vi "GetServerVIName.vi"(1 "ROS":T1={"topic port"=0, "Node"="", "topic"="", "type"="", "node port"=0, "error "={"status"=FALSE, "code"=0, "source"=""}, "Direction"=enum."Node", "Update (ms)"=1, "FIFO size"=1}) -> (0 "vi name":string)   [LabVIEW 2015]
doc: "Gets VI name"
uses:
  _ROSControl.ctl
  _ROSDirection.ctl
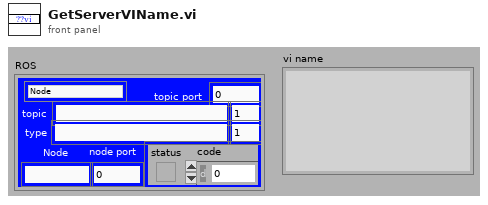
[diagram p1: front panel]
types:
  T1 = typedef "_ROSControl.ctl" = cluster{"topic port":u16, "Node":string, "topic":string, "type":string, "node port":u16, "error ":errorcluster, "Direction":T2, "Update (ms)":u16, "FIFO size":u16}
  T2 = typedef "_ROSDirection.ctl" = enum16{"Node", "Publisher", "Subscriber", "ServiceClient", "ServiceProvider"}
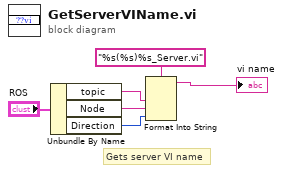
[diagram p0: block diagram]
diagram:
  # "Gets server VI name"
  n1 = Unbundle By Name("ROS") -> ("topic"=w3:string, "Node"=w2:string, "Direction"=w4:T2)
  n2 = Format Into String(format string="%s(%s)%s_Server.vi", w3, w2, w4) -> (resulting string=→"vi name":string)  [unwired: 2 in, 1 out]
